vi "Write Single Coil.vi"(7 "unit ID":u8, 8 "error in":errorcluster, 9 "coil to write":bool, 10 "address":u16, 11 "Modbus slave in":refnum<class "Modbus Slave.lvclass">) -> (0 "error out":errorcluster, 3 "Modbus slave out":refnum<class "Modbus Slave.lvclass">)   [LabVIEW 2013, in "Modbus Library - Advance.lvlib" / "Modbus Slave.lvclass"]
doc: "Writes <B>coil to write</B> to <B>address</B> of the device."
uses:
  Modbus Slave.lvclass
  Modbus Slave.lvclass/Modbus Slave.ctl
  Standard Data Model/Standard Data Model.lvclass
  Super Data Model/Super Data Model.lvclass
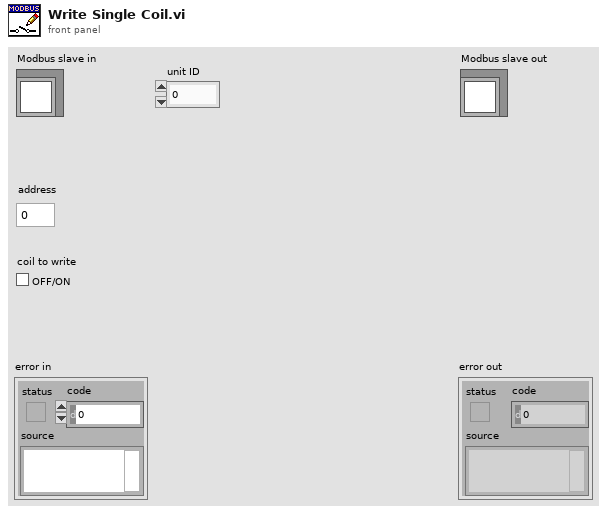
[diagram p1: front panel]
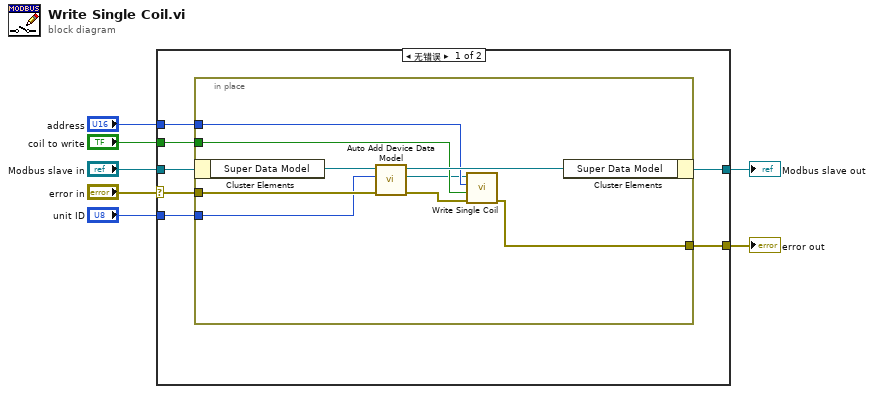
[diagram p0: block diagram]
diagram:
  n1 = case shown="无错误" "error in" {
    selector: "error in" -> [w10 w25]
    tunnel: [w8 w25] -> w6
    tunnel: "Modbus slave in" -> [w12 w24]
    tunnel: "coil to write" -> [w14 _]
    tunnel: "address" -> [w13 _]
    tunnel: [w11 w24] -> w2
    tunnel: "unit ID" -> [w9 _]
    frame No Error {
      n2 = in-place {
        in-place-border: w14 -> [w18]
        in-place-border: w13 -> [w19]
        in-place-border: w10 -> [w22]
        in-place-border: w9 -> [w21]
        in-place-border: [w17] -> w8
        n3 = in-place-cluster #1(w12) -> ("Super Data Model"=w23:refnum<class "Super Data Model.lvclass">)
        n4 = call "Auto Add Device Data Model.vi"("error in"=w22, "unit ID"=w21, "Super Data Model in"=w23) -> ("error out"=w16:errorcluster, "device data model"=w15:refnum<class "Standard Data Model.lvclass">, "Super Data Model out"=w20:refnum<class "Super Data Model.lvclass">)  [unwired: 6 in]
        n5 = call-dynamic "Write Single Coil.vi"("error in"=w16, "coil value"=w18, "address"=w19, "device data model in"=w15) -> ("error out"=w17:errorcluster)  [unwired: 6 in, 1 out]
        n6 = in-place-cluster #1("Super Data Model"=w20) -> (w11:refnum<class "Modbus Slave.lvclass">)
      }
    }
    frame Error {
    }
  }
  "error out" <- w6
  "Modbus slave out" <- w2
